vi "VI실행.vi"() -> ()   [LabVIEW 2014]
panel:
  in  "vi 경로":path
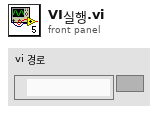
[diagram p1: front panel]
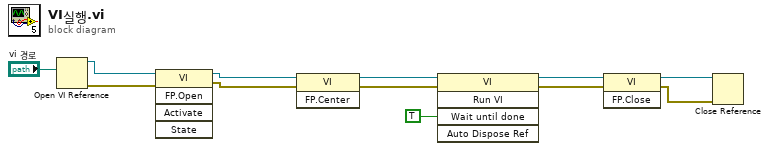
[diagram p0: block diagram]
diagram:
  n1 = Open VI Reference(vi path="vi 경로") -> (vi reference=w11:refnum<vi>, error out=w10:errorcluster)  [unwired: 5 in]
  n2 = invoke class="VI" method="FP.Open"(reference=w11, error in=w10) -> (reference out=w9:refnum<vi>, error out=w8:errorcluster)  [unwired: 3 in, 3 out]
  n3 = invoke class="VI" method="FP.Center"(reference=w9, error in=w8) -> (reference out=w7:refnum<vi>, error out=w6:errorcluster)  [unwired: 1 in, 1 out]
  n4 = invoke class="VI" method="Run VI"(reference=w7, error in=w6, "Wait until done"=TRUE ("완료될 때까지 기다림")) -> (reference out=w4:refnum<vi>, error out=w3:errorcluster)  [unwired: 2 in, 3 out]
  n5 = invoke class="VI" method="FP.Close"(reference=w4, error in=w3) -> (reference out=w2:refnum<vi>, error out=w1:errorcluster)  [unwired: 1 in, 1 out]
  n6 = Close Reference(reference=w2, error in (no error)=w1) -> ()  [unwired: 1 out]
